vi "Create Server SMO.vi"(6 "Debug Mode?":bool, 8 "error in (no error)":errorcluster, 9 "Commands":string[](array[string]), 10 "Port":u16, 11 "RemoteControl in":refnum<class "RemoteControl.lvclass">) -> (0 "error out":errorcluster, 3 "RemoteControl out":refnum<class "RemoteControl.lvclass">)   [LabVIEW 2019, in "RemoteControl.lvclass"]
uses:
  RemoteControl.lvclass
  <vilib>/JKI/JKI SMO/SMO/SMO.lvclass
  Typedefs/RC Process Type--Enum.ctl
  <vilib>/JKI/JKI SMO/SMO/Typedefs/SMOState --Enum.ctl
  <vilib>/JKI/JKI SMO/SMO/Typedefs/Reserve State--Enum.ctl
  <vilib>/JKI/JKI SMO/SMO/Typedefs/Public Events.ctl
  Typedefs/Message--Cluster.ctl
  Typedefs/PublicEvents--RemoteControl.SendMessageFromProcess.ctl
  Typedefs/PublicEvents--Cluster.ctl
  <userlib>/LevyLab/Configuration/Debug.lvlib
  <userlib>/LevyLab/Configuration/subsystems/Attribute.Debug/DebugBehavior.ctl
  <userlib>/LevyLab/Configuration/subsystems/Attribute.Debug/Attribute.Debug.lvclass
  C:/Program Files (x86)/National Instruments/LabVIEW 2019/vi.lib/JKI/JKI SMO/SMO/SMO.lvclass
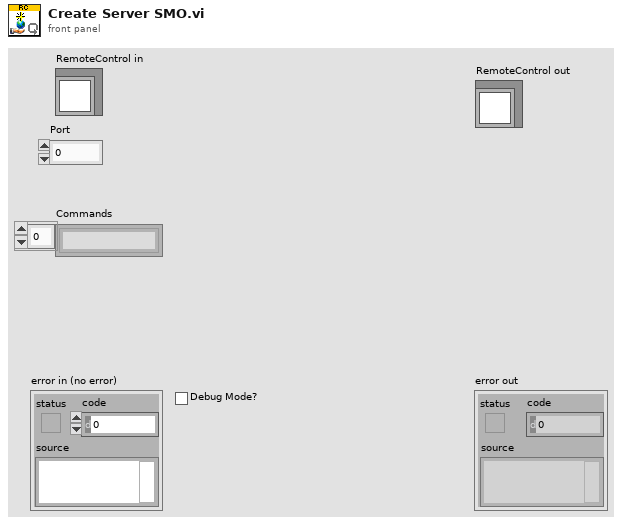
[diagram p1: front panel]
types:
  T1 = typedef "Debug.lvlib/Attribute.Debug.lvclass/DebugBehavior.ctl" = enum16{"Normal", "Debug"}
  T2 = typedef "RemoteControl.lvclass/RC Process Type--Enum.ctl" = enum16{"Listener", "Server", "Client"}
  T3 = typedef "RemoteControl.lvclass/PublicEvents--Cluster.ctl" = cluster{"SendMessageFromProcess":refnum<user-event>}
  T4 = typedef "smo.lvlib/SMO.lvclass/Public Events.ctl" = cluster{"Error":refnum<user-event>, "State":refnum<user-event>, "Reserve State":refnum<user-event>}
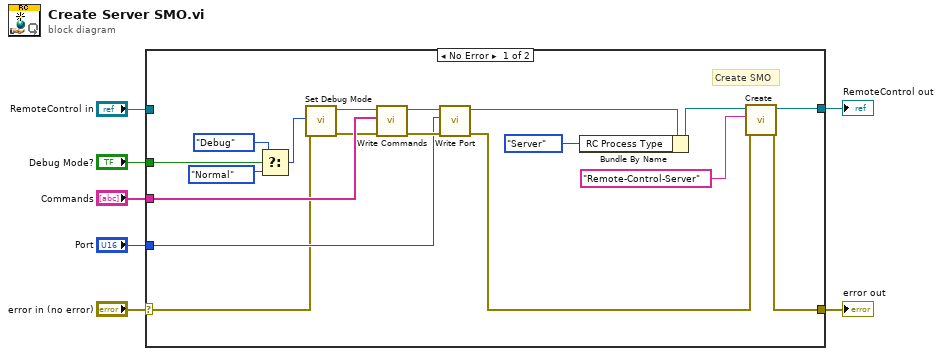
[diagram p0: block diagram]
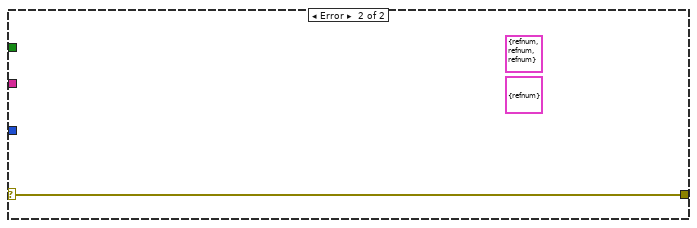
[diagram p2: hidden frame]
diagram:
  n1 = case shown="No Error" "error in (no error)" {
    selector: "error in (no error)" -> [w8 w26]
    tunnel: [w24 w26] -> w6
    tunnel: [w25 _] -> w5
    tunnel: "Commands" -> [w17 _]
    tunnel: "Port" -> [w16 _]
    tunnel: "RemoteControl in" -> [_ _]
    tunnel: "Debug Mode?" -> [w9 _]
    frame No Error {
      # "Create SMO"
      n2 = Select(t=DebugBehavior."Debug" ("Behavior"), s=w9, f=DebugBehavior."Normal" ("Behavior")) -> (s? t:f=w10:T1)
      n3 = call <userlib>:"Set Debug Mode.vi"("error in (no error)"=w8, "Behavior"=w10) -> ("error out"=w13:errorcluster, "SMO out"=w14:refnum<class "SMO.lvclass">)  [unwired: 8 in]
      n4 = call-dynamic "Write Commands.vi"("error in (no error)"=w13, "Commands"=w17, "RemoteControl in"=w14) -> ("error out"=w20:errorcluster, "RemoteControl out"=w19:refnum<class "RemoteControl.lvclass">)  [unwired: 7 in]
      n5 = call-dynamic "Write Port.vi"("error in (no error)"=w20, "Port"=w16, "RemoteControl in"=w19) -> ("error out"=w18:errorcluster, "RemoteControl out"=w15:refnum<class "RemoteControl.lvclass">)  [unwired: 7 in]
      n6 = Bundle By Name(cluster=w15, "RC Process Type"=RC_Process_Type--Enum."Server") -> (w22:refnum<class "RemoteControl.lvclass">)
      n7 = call <vilib>:"Create.vi"("error in (no error)"=w18, "Subsystem Name (optional)"="Remote-Control-Server" ("format string"), "SMO"=w22) -> ("error out"=w24:errorcluster, "SMO out"=w25:refnum<class "RemoteControl.lvclass">)  [unwired: 6 in, 1 out]
    }
    frame Error {
      (unwired) T3 {"SendMessageFromProcess"=refnum} ("RC Public Events")
      (unwired) T4 {"Error"=refnum, "State"=refnum, "Reserve State"=refnum} ("Public Events")
    }
  }
  "error out" <- w6
  "RemoteControl out" <- w5
